vi "HFRR ADV v012 new software.vi"() -> ()   [LabVIEW 2025]
uses:
  <vilib>/picture/picture.llb/imagedata.ctl
  src/Support Vi/Auto Start enum.ctl
  src/CAMERA CODE/CAMERA LIVE FEED ENUM.ctl
  src/CAMERA CODE/POST ANALYSIS ENUM.ctl
  <vilib>/Utility/NIReport.llb/HTML Report Image Alignment.ctl
  9464fbe3-7a28-44f6-aba5-8c8738b059c4.vi
  65798b11-504e-4bc8-a248-6a605d2bfeff.vi
  e8a7d01f-49de-42c3-94d4-2c8624f58f4e.vi
  5efb8110-29bd-47d9-92d0-c4703c9d257e.vi
  c311699a-12ba-46ef-ac8f-427021fdbf06.vi
  b1c79803-6f73-4462-b675-f7b5eb88be7c.vi
  62610586-f3e3-47d7-ba3d-7d74a0c80884.vi
  25e8caaf-84ea-468e-9ff7-adb0e8b96af1.vi
  63a25930-3a94-42f5-b8a7-a5485c4ba60b.vi
  865355ac-209e-4fc1-945d-f9c41f79343a.vi
  8bf3357a-fd86-4b15-a53b-ddd460c8ef7b.vi
  8955922f-f541-41b3-8336-ee15e0ce1609.vi
  <vilib>/numeric/Random Number (Range) DBL.vi
  <vilib>/Analysis/baseanly.llb/Mean (DBL).vi
  <vilib>/Utility/error.llb/Trim Whitespace One-Sided.vi
  <vilib>/Instr/_visa.llb/VISA Configure Serial Port (Instr).vi
  Instance          10 41Saved   WinDucom--std ed hfrr-WO 2464 v02 .vi
  <vilib>/addons/control/pid/pid.llb/PID (DBL).vi
  Instance          23 41Saved   WinDucom--std ed hfrr-WO 2464 v02 .vi
  <vilib>/Utility/NIReport.llb/Append Image to Report (path wrap).vi
  <vilib>/printing/OpenHTMLReport.llb/Open HTML Report in Browser (Refnum).vi
  <vilib>/Utility/NIReport.llb/Append Report Text (str wrap).vi
  Instance          11 41Saved   WinDucom--std ed hfrr-WO 2464 v02 .vi
  Instance           6 41Saved   WinDucom--std ed hfrr-WO 2464 v02 .vi
  <vilib>/Utility/NIReport.llb/NI_report.lvclass
  <vilib>/addons/control/pid/NI_PID_pid.lvlib
  Instance          22 41Saved   WinDucom--std ed hfrr-WO 2464 v02 .vi
  Instance          25 41Saved   WinDucom--std ed hfrr-WO 2464 v02 .vi
  <vilib>/NI Modbus.llb/MB Serial Master Query Read Input Registers (poly).vi
  Instance          35 41Saved   WinDucom--std ed hfrr-WO 2464 v02 .vi
  Instance          38 41Saved   WinDucom--std ed hfrr-WO 2464 v02 .vi
  <vilib>/Utility/NIReport.llb/NI_ReportGenerationCore.lvlib
  <vilib>/Analysis/NI_AALPro.lvlib
  <vilib>/Analysis/NI_AALBase.lvlib
  kernel32.dll
  <vilib>/measure/NI_MABase.lvlib
  <vilib>/NI Modbus.llb/MB Serial Master Query Write Single Register (poly).vi
  <vilib>/ptbypt/NI_PtbyPt.lvlib
panel:
  out "Status":dbl[](array[numeric])
  out "Calibrated Voltage Value":dbl[](array[numeric])
  out "1D stroke":dbl[](array[numeric])
  out "Calibration 1.2":dbl
  out "Calibration 1.0":dbl
  out "Calibration 0.8":dbl
  out "Calibration 0.6":dbl
  out "Calibration 0.4":dbl
  out "Calibration 0.2":dbl
  out "LVDT STROKE  Calibration":dbl
  in  "Continue Stroke step 9":bool
  in  "Step 7 Back":bool
  out "Boolean":bool
  out "Read Humidity":string
  out "LVDT STROKE":dbl
  out "AmbRaw":dbl
  out "SampleRaw":dbl
  out "Kd":dbl
  out "Ki":dbl
  out "Kp":dbl
  out "Active Error Code":dbl
  out "Vpp":dbl
  out "Dac Status":dbl
  out "Ambient Temperature":dbl
  out "Current Duty Cycle":dbl
  out "Target Sample Temperature":dbl
  out "Sample Temperature":dbl
  in  "Add up Stroke":dbl=0.03
  out "START TEMP":bool
  in  "Command":string
  out "Due read":string
  out "UNI READ":string
  in  "STROKE":dbl[](array[numeric])=[0.1, 0.2, 0.3, 0.4, 0.5, 0.6, 0.7, 0.8, 0.9, 1.0, 1.1, 1.2]
  in  "1,2":dbl=1.1278
  in  "1.1":dbl=1.0761
  in  "1.0":dbl
  in  "0.9":dbl=0.9543
  in  "0.8":dbl
  in  "0.7":dbl=0.8122
  in  "0.6":dbl
  in  "0.5":dbl=0.639
  in  "0.4":dbl=0.5425
  in  "0.3":dbl=0.4226
  in  "0.2":dbl=0.2961
  in  "0.1":dbl=0.1677
  in  "calibration values":dbl[](array[numeric])=[0.1677, 0.2961, 0.4226, 0.5425, 0.639, 0.737, 0.8122, 0.864, 0.9543, 1.0177, 1.0761, 1.1278]
  out "prev_vc_cmd":dbl
  out "integral_accumulator_in":dbl
  out "prev_error":dbl
  in  "startup_cmd":dbl=400.0
  in  "min_amplitude":dbl
  in  "max_amplitude":dbl=1300.0
  in  "max_step_change":dbl=45.0
  in  "kd":dbl=40.0
  in  "ki":dbl=300.0
  in  "kp":dbl=1000.0
  in  "dt":dbl=0.05
  out "output Vpp":dbl
  out "error out 9":errorcluster
  out "LVDT MIN":dbl
  out "LVDT MAX":dbl
  out "LVDT Peak":dbl
  out "pizo raw":dbl
  out "Friction":dbl
  out "cof 2":dbl
  in  "main tab sub":enum32{"Page 1", "Page 2"}(tab)
  out "About":cluster{"About Display":string}={"About Display"="Software Version : Lab IQ\\WO 2472\\ v02\n\nRelease Period    : May 2026  "}
  in  "Info":bool
  in  "Quit":bool
  out "Humidity Port":bool=TRUE caption="Port 2"
  out "Standard 2":string="ASTM D6079 TEST CONDITIONS"
  out "powstat":bool caption="Power Status"
  out "Test \nStatus":bool caption="Test Status"
  out "Port 3":bool=TRUE caption="Port 1"
  out "Port 1a":bool caption="Port 1 a"
  out "Port 4":bool=TRUE caption="Port 2"
  out "Port 2a":bool caption="Port 2 a"
  in  "Main Dashboard Buttons":T1(radio) caption="Radio Buttons - Customizable"
  out "Time Stamp":string
  in  "Main Tab":T2(tab)
  out "Service Password Log":string="Incorrect Password"
  in  "Password 3":cluster{"Service Password":string}
  in  "Headen Service Button":bool
  in  "Sign In":bool
  in  "USER ID":string
  in  "USERNAME":string
  out "Auto Scar Check":cluster{"String 2":string}
  in  "Calibration":bool
  in  "Auto":bool
  in  "test time":dbl=75.0 caption="TEST DURATION" min=1.0 max=75.0 step=1.0
  in  "Set Rh":dbl=53.0 caption="HUMIDITY" min=53.0 max=53.0 step=1.0
  in  "Set Temp":dbl=60.0 caption="TEMPERATURE" min=40.0 max=150.0 step=1.0
  in  "Set Strk":dbl=1.0 caption="STROKE LENGTH" min=1.0 max=1.0 step=1.0 format="%.3f"
  in  "NORMAL LOAD":dbl=2.0 caption="APPLIED LOAD" min=1.0 max=10.0 step=1.0
  in  "Set Hz":dbl=50.0 caption="FREQUENCY" min=50.0 max=50.0 step=50.0 format="%.1f"
  out "Standard":string="ASTM D6079 TEST CONDITIONS"
  in  "FILE":string caption="FILE NAME"
  in  "Fuel Discription :":string caption="FLUID DESCRIPTION"
  in  "Batch Ref Num :":string caption="BATCH REF NO"
  in  "Remarks :":string caption="REMARKS"
  in  "tested by":string caption="TESTED BY"
  in  "Operator ID":string caption="OPERATOR ID"
  in  "TEST STANDARD":T3(ring)
  in  "Save & Continue":bool
  in  "Calibration 2":enum32{"Main", "Page 2"}(tab)
  in  "Cal Password":string
  out "Wrong Password":string="Wrong Password Entered"
  out "Time Remaining":dbl min=0.0 max=6000.0 step=0.01 format="%<%M:%S>t"
  in  "EVENT LOG":string="4:36:36 PM       Temperature trip enabled\n4:59:03 PM       Test started  — ASTM D6079-25"
  in  "Single/Multiple":enum32{"Single ", "Multiple"}(radio)=enum."Multiple" caption="Radio Buttons - Customizable"
  in  "Single - Graph":u16(ring) items=["Co-efficient of Friction", "Frictional Force ( N )", "ECR ( % )", "Temperature ( Deg C )", "Humidity ( %RH )", "Stroke ( mm )"]
  in  "Num/Graph":enum32{"Numeric Display", "Graph Display"}(radio) caption="Radio Buttons - Customizable"
  in  "Reset Graph":bool
  in  "Main Tab Display":T4(tab)
  out "COF 3":dbl min=0.0 max=1.0 step=0.001 format="%.3f"
  out "measured_stroke":dbl format="%.3f"
  in  "FRICVALZ 4":bool
  out "Set Stroke:":dbl
  out "Set Frequency:":dbl
  out "Set Humidity:":dbl
  out "Set Temperature:":dbl
  in  "Humidity":bool
  out "Horizontal Slider Control":dbl(slide) min=0.0 max=100.0 scale=0.0..75.0
  in  "Heater Button":bool
  out "HEATER":bool
  out "Humidity ( %RH )":dbl caption="Humidity 3" format="%.1f"
  out "AIR TEMP":dbl caption="Air Temperature  ( °C )" min=0.0 max=150.0 step=1.0 format="%.1f"
  out "Frequency ( Hz )":dbl=50.0 caption="Frequency" min=10.0 max=250.0 step=0.1 format="%.2f"
  out "Stroke 2":dbl=1.0 caption="Stroke" format="%.3f"
  out "TEMP":dbl min=0.0 max=150.0 step=1.0 format="%.1f"
  out "ecr 3":dbl min=0.0 max=100.0 step=1.0
  out "FF 3":dbl min=0.0 max=12.0 step=0.01 format="%.3f"
  out "Hum":dbl=34.66389660208565 min=0.0 max=150.0 step=1.0
  out "Stroke 4":dbl=1.0 caption="Stroke" format="%.3f"
  out "Stroke ( mm )":cluster{"y":dbl, dbl, "y":dbl}(graph) caption="Waveform Chart - Light"
  out "Humidity ( %RH )":dbl(graph) caption="Waveform Chart - Light"
  out "Status 13":bool
  in  "Set Temp 2":dbl=65.0 caption="TRIP" min=20.0 max=150.0 step=1.0
  in  "trip1 8":bool
  in  "FRICVALZ 2":bool
  out "COF 2":dbl min=0.0 max=1.0 step=0.001 format="%.3f"
  out "Coefficient of Friction":dbl(graph) caption="Waveform Chart - Light"
  out "Electrical Contact Resistance ( % )":dbl(graph) caption="Waveform Chart - Light"
  out "FF 2":dbl min=0.0 max=12.0 step=0.01 format="%.3f"
  out "Frictional Force ( N )":dbl(graph) caption="Waveform Chart - Light"
  out "TEMP 2":dbl=34.66389660208565 min=0.0 max=150.0 step=1.0
  out "Temperature ( Deg C )":dbl(graph) caption="Waveform Chart - Light"
  out "Single":T5(tab)
  out "COF 4":dbl min=0.0 max=1.0 step=0.001 format="%.3f"
  out "Coefficient of Friction":dbl(graph) caption="Waveform Chart - Light"
  out "FF 4":dbl min=0.0 max=12.0 step=0.01 format="%.3f"
  in  "FRICVALZ 3":bool
  out "Frictional Force ( N )":dbl(graph) caption="Waveform Chart - Light"
  out "Electrical Contact Resistance ( % )":dbl(graph) caption="Waveform Chart - Light"
  out "TEMP 3":dbl=34.66389660208565 min=0.0 max=150.0 step=1.0
  out "Temperature ( Deg C )":dbl(graph) caption="Waveform Chart - Light"
  out "Hum 2":dbl=34.66389660208565 min=0.0 max=150.0 step=1.0
  out "Humidity ( %RH )":dbl(graph) caption="Waveform Chart - Light"
  out "Stroke 3":dbl=1.0 caption="Stroke" format="%.3f"
  out "Stroke ( mm )":cluster{"y":dbl, dbl, "y":dbl}(graph) caption="Waveform Chart - Light"
  out "Test Duration Display":string
  in  "Test Duration Status":dbl(slide) scale=0.0..100.0
  in  "RUN":bool
  in  "Auto Start Test":bool caption="RUN"
  out "Auto Scar Check  2":cluster{"String 2":string}
  in  "Magnification len live scar":string(combo)="5x" caption="MAGNIFICATION LEVEL"
  in  "FILE 3":string(combo) caption="FILE NAME"
  in  "SCAR MEASURMENT":enum32{"Auto Scar", "Manual Scar"}(radio)=enum."Manual Scar" caption="Radio Buttons - Customizable"
  in  "Cap Live Image":bool caption="Save Image"
  out "Zoom Factore":dbl format="%#.0f"
  in  "OUT":bool
  in  "In":bool
  in  "Confirm Measrurement":bool
  in  "Magnification :":string(combo)="5x"
  in  "Open Image":bool
  in  "Test File List :":string(combo)
  in  "Calibration Tab":enum32{"Measrument", "Calibrate"}(tab)
  out "Major Axis":dbl
  out "Minor Axis":dbl
  out "Average":dbl
  in  "Back Square":bool
  out "10x Gain":dbl
  out "5x Gain":dbl
  in  "Actual (µm)":dbl=1.0 caption="Actual (mm)" format="%.6f"
  out "Measurment (mm)":dbl caption="mm" format="%.3f"
  in  "Save Change":bool caption="Save Cal"
  in  "change Gain":bool
  in  "Calibrate":bool
  in  "Resize Tool":bool
  in  "Fit to Screen Tool":bool
  in  "ROI Color Tool":bool
  in  "Clear ROI Tool":bool
  in  "Rectangle Tool":bool
  in  "Pan Tool":bool
  in  "line tool":bool
  in  "Frequency":bool
  in  "Sample Temperature":bool
  in  "Stroke":bool
  in  "Humidity":bool
  in  "Air Temperature":bool
  in  "Tab Control 2":T6(tab)=enum."Humidity"
  in  "rstv2":bool
  out "Coefficient Of Friction":cluster{dbl[], dbl[]}[](graph)
  out "КОФ1":dbl caption="COF1 :" min=0.0 max=200.0 step=0.1 format="%.3f"
  out "КОФ2":dbl caption="COF2 :" min=0.0 max=200.0 step=0.1 format="%.3f"
  out "КОФ3":dbl caption="COF3 :" min=0.0 max=200.0 step=0.1 format="%.3f"
  out "КОФ4":dbl caption="COF4 :" min=0.0 max=200.0 step=0.1 format="%.3f"
  in  "RSTV1 3":bool
  out "Air Temperature  ( °C )":cluster{dbl[], dbl[]}[](graph)
  in  "RSTV1 2":bool
  out "Humidity ( %RH )":cluster{dbl[], dbl[]}[](graph)
  in  "RSTV1 4":bool
  out "Stroke ( mm )":cluster{dbl[], dbl[]}[](graph)
  out "КОФ2 5":dbl caption="Stroke 4 :" min=0.0 max=200.0 step=0.1 format="%.3f"
  out "КОФ2 4":dbl caption="Stroke 3 :" min=0.0 max=200.0 step=0.1 format="%.3f"
  out "КОФ2 3":dbl caption="Stroke 2 :" min=0.0 max=200.0 step=0.1 format="%.3f"
  out "КОФ2 2":dbl caption="Stroke 1:" min=0.0 max=200.0 step=0.1 format="%.3f"
  out "CP2":dbl=nan min=0.0 max=200.0 step=0.1 format="%.3f"
  out "CP1":dbl=nan min=0.0 max=200.0 step=0.1 format="%.3f"
  in  "RST CP":bool
  out "Sample Temperature ( °C )":cluster{dbl[], dbl[]}[](graph)
  in  "RST CP 2":bool
  out "XY Graph 13":cluster{dbl[], dbl[]}[](graph)
  out "Frequency ( Hz )":cluster{dbl[], dbl[]}[](graph)
  in  "RST CP 3":bool
  out "Air Temp ( °C ) vs Humidity ( % RH )":cluster{dbl[], dbl[]}[](graph)
  in  "OPEN 1":bool
  out "String Control 2":string="  "
  out "String Control":string
  out "String Control 7":string
  in  "OPEN 4":bool
  out "String Control 8":string=" "
  in  "OPEN 2":bool
  out "String Control 3":string
  out "String Control 4":string=" "
  in  "OPEN 3":bool
  out "String Control 6":string=" "
  out "String Control 5":string
  in  "Coefficient Of Friction":bool
  in  "OPEN":bool
  in  "Main Calibration Tab":T7(tab)
  in  "Calibration Selection":T8(radio) caption="Radio Buttons - Customizable"
  in  "Main Stroke Tab":T9(tab)
  in  "Continue Stroke":bool
  in  "Back Stroke":bool
  in  "Step 2 Back":bool
  in  "Continue Stroke step 2":bool
  in  "Step 3 Back":bool
  in  "Continue Stroke step 3":bool
  in  "Step 4 Back":bool
  in  "Continue Stroke step 4":bool
  in  "Step 5 Back":bool
  in  "Continue Stroke step 5":bool
  in  "Step 6 Back":bool
  in  "Continue Stroke step 6":bool
  in  "Back Stroke step 7":bool
  in  "Continue Stroke step 7":bool
  in  "Stroke Test Complete":T10(tab)
  out "MOVE CARRIAGE TO":dbl caption="mm" format="%.1f"
  out "1.2":bool
  out "1.0 2":bool
  out "0.8 2":bool
  out "0.6 2":bool
  out "0.4 2":bool
  out "0.2 2":bool
  out "0.2mm":bool
  out "0.4 mm":bool
  out "0.6 mm":bool
  out "0.8mm":bool
  out "1.0 mm":bool
  out "1.2 mm":bool
  in  "Back Stroke step 8":bool
  in  "Continue Stroke step 8":bool
  in  "Back Stroke 8":bool
  in  "Accept & Save":bool
  out "Point 6 - 1.2 mm":bool caption="CONFIRMED"
  out "Point 5 - 1.0 mm":bool caption="CONFIRMED"
  out "Point 4 - 0.8 mm":bool caption="CONFIRMED"
  out "Point 3 - 0.6 mm":bool caption="CONFIRMED"
  out "Point 2 - 0.4 mm":bool caption="CONFIRMED"
  out "Point 1 - 0.2 mm":bool caption="CONFIRMED"
  in  "Tab Control 5":T11(tab)
  in  "message":string="*Entered password is wrong"
  in  "Password 2":string caption="Password (Advance Setting)"
  in  "EDIT 2":bool
  in  "Language Selection":enum16{"English", "Russian"}(ring)
  in  "SrvM CP 2":bool caption="Reset calibrate\n password"
  in  "SrvM CP":bool caption="Reset calibrate\n password"
  in  "Password":string
  in  "SAVE":bool
  in  "File Path":path=path "C:/LAB-IQ-NXT 2010/1582/1582" caption="File path"
  in  "EDIT":bool
  out "AIR TEMPERATURE  Calibration Error":dbl=1.0 caption="Air Temperature :" min=0.0001 max=100.0 step=0.0001
  out "TEMPERATURE  Calibration Error":dbl=1.0 caption="Temperature :" min=0.0001 max=100.0 step=0.0001
  out "HUMIDITY  Calibration Error":dbl=1.0 caption="Humidity :"
  out "DISPLACEMENT  Calibration Error":dbl=1.0255 caption="Displacement :"
  out "STROKE Calibration Error":dbl=700.0 caption="Stroke Gain :"
  out "FRIC. FORCE Calibration Error":dbl=3.7633 caption="Frictional Force :" min=0.0001 max=100.0 step=0.0001
  in  "AIR TEMP INTERCEPT: 2":dbl=-2.9906 caption="Air Temperature Intercept:" format="%.4f"
  in  "AIR TEMP INTERCEPT:":dbl caption="Air Temperature Intercept :" format="%.4f"
  in  "TEMP INTERCEPT: 2":dbl=-2.9906 caption="Temperature Intercept :" format="%.4f"
  in  "TEMP INTERCEPT:":dbl caption="Temperature Intercept :" format="%.4f"
  in  "AIR TEMPERATURE : 2":dbl=57.9984 caption="Air Temperature :" min=0.0001 max=100.0 step=0.0001 format="%.4f"
  in  "AIR TEMPERATURE :":dbl=1.0 caption="Air Temperature :" min=0.0001 max=100.0 step=0.0001 format="%.4f"
  in  "TEMPERATURE : 2":dbl=57.9984 caption="Temperature :" min=0.0001 max=100.0 step=0.0001 format="%.4f"
  in  "TEMPERATURE :":dbl=1.0 caption="Temperature :" min=0.0001 max=100.0 step=0.0001 format="%.4f"
  in  "HUMIDITY: 2":dbl=1.0 caption="Humidity :" min=0.95 max=1.05 step=0.001 format="%.2f"
  in  "HUMIDITY:":dbl=1.0 caption="Humidity :" min=0.95 max=1.05 step=0.01 format="%.2f"
  in  "DISPLACEMENT : 4":dbl=0.88 caption="Displacement :" min=0.5 max=1.8 step=0.01 format="%#.2f"
  in  "DISPLACEMENT :":dbl=1.0255 caption="Displacement :"
  in  "STROKE GAIN : 2":dbl=900.0 caption="Stroke Gain :" min=500.0 max=1500.0 format="%#.1f"
  in  "STROKE GAIN :":dbl=700.0 caption="Stroke Gain :"
  in  "FRIC. FORCE : 2":dbl=1.0 caption="Frictional Force :" min=0.95 max=1.05 step=0.0001 format="%.2f"
  in  "FRIC. FORCE :":dbl=3.7633 caption="Frictional Force :" min=0.0001 max=100.0 step=0.0001 format="%.4f"
  in  "Tab Control 7":T12(tab)
  in  "S.NO":string="1333"
  in  "Standard Slip Gauge (mm)":dbl
  out "String 26":string="Rh"
  out "String 13":string="Rh"
  out "String 5":string="N"
  out "String 3":string="Hz"
  out "Time slide":dbl(slide)=70.0 scale=0.0..2500.0
  in  "ENTER THE NEW PASSWORD":string caption="Enter The New Password"
  in  "ENTER CURRENT PASSWORD":string caption="Enter Current Password"
  in  "Camera Port :":string(combo)="cam0"
  in  "C3 :":refnum<visa-resource-name>="COM8"
  out "Port 2 Error":errorcluster={"status"=TRUE, "code"=-1073807343, "source"="Property Node (arg 1) in VISA Configure Serial Port (Instr).vi->Winducom 2010--std ed hfrr-wo1768-V18.vi"}
  out "Port 1 Error":errorcluster={"status"=TRUE, "code"=-1073807343, "source"="Property Node (arg 1) in VISA Configure Serial Port (Instr).vi->Winducom 2010--std ed hfrr-wo1768-V18.vi"}
  in  "CH-HUMIDITY DRY":u16=3 caption="Ch-Humidity Wet:" max=7 step=1
  in  "CH-HUMIDITY WET":u16=4 caption="Ch-Humidity Dry:" max=7 step=1
  in  "CH-HEATER":u16=2 caption="Ch-Heater:" max=7 step=1
  in  "CH-POWER -":u16=1 caption="Ch-Power -:" max=7 step=1
  in  "CH-POWER +":u16 caption="Ch-Power +:" max=7 step=1
  out "String 4":string
  in  "Prog Due":bool
  in  "Prog Uno":bool
  in  "Com Port 2":refnum<visa-resource-name>="COM7" caption="C2 :"
  in  "Com Port 1":refnum<visa-resource-name>="COM5" caption="C1 :"
  in  "SAVE 2":bool
  in  "Additional Parameter":T13(tab)
  out "CAMERA ROI MIN TEMP":bool
  in  "CAMERA ROI MAX TEMP":bool
  out "LIVE FEED MIN TEMP":bool
  in  "LIVE FEED MAX TEMP":bool
  in  "Temperature Off Command":bool
  in  "Temperature On Command":bool
  in  "Humidity Off Command":bool
  in  "Humidity On Command":bool
  out "Elapsed time":dbl caption="Elapsed Time" min=0.0 max=6000.0 step=0.01 format="%.2f"
  in  "Remaining Time":dbl min=0.0 max=180000.0 step=0.0001 format="%<%H:%M:%S>t"
  out "Auto Start Temp":bool
  out "Auto stop temp":bool
  in  "TestCompFlg":bool
  out "StartFlg":bool
  in  "Start Time":bool
  in  "sign in temp":bool
  in  "manual temp log":bool
  in  "Reach point temp":bool
  in  "Manual Humididty Reached":bool
  out "Humidity temp":dbl
  in  "Test ID":string
  in  "Reach point Humidity":bool
  in  "error in (no error) 2":errorcluster
  out "Instrument Status":bool=TRUE caption="Load COM Status"
  in  "Heater Trip Temp":bool
  out "String 41":string=":-@(Paltro : HIGH FREQUENCY RECIPROCATORY TEST RIG    DEFINITON FILE )      "
  out "Service Password enable":bool
  out "TEST FILE NAM,E SAVED":bool
  out "error out 6":errorcluster
  out "error out 7":errorcluster
  out "error out 8":errorcluster
  in  "Ambient Humidity :":dbl format="%.1f"
  out "Camera List":string
  out "Image path  2":path caption="selected path"
  out "100x gain":dbl
  out "Pixel Value":dbl
  in  "Enum - Selector":T14
  out "Image path":path
  out "Error":errorcluster={"status"=TRUE, "code"=-1073807343, "source"="Property Node (arg 1) in VISA Configure Serial Port (Instr).vi->Winducom 2010--std ed hfrr-wo1768-V18.vi"}
  out "Bytes at Humidity Port":dbl
  in  "Com Port 4":refnum<visa-resource-name>="COM7" caption="COM Port Humidity :"
  in  "String 11":string
  in  "WriteHumidity":string[](array[string])
  out "LastCom":string
  in  "Write S":bool
  out "STALL :":string
  out "CURRENT :":string
  out "DEHUM :":string
  out "FAN_OUT :":string
  out "FAN_IN :":string
  out "PUMP :":string
  out "AMB_T :":string
  out "AMB_RH :":string
  out "T :":string
  out "RH :":string
  out "SET :":string
  out "STATE :":string
  out "RH Numeric:":dbl
  out "COM Status":bool=TRUE caption="Load COM Status"
  in  "Tab Control 6":enum32{"Data", "Sensor"}(tab)=enum."Sensor"
  out "Respose From Server":string
  out "standard output":string
  out "SinglePoint":string
  in  "JSON Check String":string="\"Stored\": true"
  in  "JSONH Check String":string="\"Stored\": true"
  out "standard output 2":string
  in  "Sensor Information":string[][](array[string])=[["Sensor Name", "Sensor Model Number", "Sensor Run time Hours", "Sensor State"], ["Normal Load Sensor", "MPF-AC20-X3U791", "", ""], ["Frictional Force Sensor", "MPF-AC20-X3U792", "", ""], ["Temperature Sensor", "MPF-AC20-X3U793", "", ""], ["Speed Sensor", "MPF-AC20-X3U794", "", ""], ["LVDT Sensor", "MPF-AC20-X3U795", "", ""], ["Vibration Sensor ", "MPF-AC20-X3U796", "", ""]]
  out "Respose From Server 2":string
  in  "Total No. of Tests":dbl
  in  "Upld AR":bool
  in  "Sensor File Name":string="JSON_Health.JSON"
  in  "Run test 3":bool
  in  "Sen.Upload Rate (s)":dbl=5.0 min=0.5 max=5.0 step=0.5 format="%.1g"
  in  "Upld AR 2":bool
  in  "Path":path=path "C:/LAB-IQ-NXT"
  in  "Data File Name":string="JSON_Single_Point.JSON"
  in  "Model No":string="MD987654325"
  in  "Serial No":string="HFRR2391"
  in  "Secret Key":string="22gKHnAGFaJhuNtaR9srYhcD6RQR8M7Zp2xk4ssPTuwGqWUBv7WxW7cXAFkFFbns"
  in  "Upload Rate (s)":dbl=1.0 min=0.5 max=5.0 step=0.5 format="%.1g"
  out "Test Standard":string
  out "error out 5":errorcluster
  out "after substring":string
  out "before substring 2":string
  in  "Temperature after test 3":dbl caption="Temp After Test" format="%#_5g"
  in  "Humidity after test 3":dbl caption="Humidity After Test" format="%#_5g"
  out "autostrtflg":bool
  out "airtempflg":bool
  out "z_measure":dbl
  out "Read String":string
  out "Waveform Graph 5":dbl[](graph)
  out "Waveform Chart 3":dbl[](graph)
  out "set temp old":dbl
  out "Error Code":errorcluster
  in  "Rd":bool
  out "String 10":string
  in  "Length 2":i16=16 caption="Set" min=1 max=60 step=1
  out "path 2":path
  out "image data":T15
  out "new picture":picture
  out "error out 2":errorcluster
  out "String Indicator 4":string
  out "String Indicator 3":string
  in  "OPEN 5":bool
  out "string1 5":string
  out "String 49":string="Tested by"
  out "String 48":string="Sample ID "
  out "String 47":string="Tested date"
  out "String 46":string="S.NO"
  out "test by 2":string
  in  "ISO : WS1.4":enum32{"Page 1", "Page 2"}(tab)
  in  "Save Results":bool
  out "String 23":string="ISO : WS1.4"
  out "Rh After":dbl min=0.0 max=100.0 step=1.0 format="%.1f"
  out "Rh Before":dbl min=0.0 max=100.0 step=1.0 format="%.1f"
  in  "Humidity before test":dbl min=0.0 max=100.0 step=1.0
  out "AVP":dbl=0.0032746494993313616 format="%.3f"
  in  "MWSD":dbl
  out "WS1.4":dbl format="%1.2f"
  in  "HCF":dbl min=0.0 max=10000.0 step=0.01 format="%.2f"
  in  "Temperature before test":dbl=1.0 caption="Temp before test" min=1.0 max=100.0 step=0.1 format="%.1f"
  in  "Humidity after test":dbl=1.0 min=1.0 max=100.0 step=1.0
  in  "Temperature after test":dbl=1.0 caption="Temp after test" min=1.0 max=100.0 step=0.1 format="%.1f"
  out "WS1.4 2":dbl caption="WS1.4" format="%#_5g"
  out "HCF 2":dbl caption="HCF" format="%#_5g"
  out "AVP 2":dbl caption="AVP" format="%#_5g"
  out "MWSD 2":dbl caption="MWSD" format="%#_5g"
  out "Temperature after test 2":dbl caption="Temp after test" format="%#_5g"
  out "Humidity after test 2":dbl caption="Humidity after test" format="%#_5g"
  out "Temperature before test 2":dbl caption="Temp before test" format="%#_5g"
  out "Humidity before test 2":dbl caption="Humidity before test" format="%#_5g"
  out "temp_@Rh sensor":string
  out "refresh flag":bool
  out "Air temp":string
  in  "hide controller":enum32{"Hidden", "controllers"}(tab)=enum."controllers"
  in  "UUID":string caption="UUID    :"
  in  "FLAG 4":dbl min=0.0 max=999999999.0 step=0.25 format="%.2f"
  out "START 3":dbl format="%.1f"
  in  "FLAG 2":dbl min=0.0 max=999999999.0 step=0.25 format="%.2f"
  out "JSON string":string
  out "Sensor Health JSON string":string
  out "run replace":bool
  out "cof":dbl caption="Frictional Torque" format="%.2f"
  out "time":dbl caption="Time \nRemaining"
  out "SEN.RUN HRS":dbl
  out "Json St Flg":bool
  out "Json End Flg":bool
  out "temp_st":string
  out "sp_st":string
  out "FF STATE":i32
  out "nlstate":string
  out "ffstate":string
  out "nl_st":string
  out "ff_st":string
  in  "in":string[](array[string])=["", "", "", "", "", "", ""]
  out "out":string[](array[string])=["Sensor State", "", "", "", "", "", ""]
  out "SinglePoint  2":string
  out "Sensor name":string[](array[string])
  out "model num":string[](array[string])
  out "run time":string[](array[string])
  out "state":string[](array[string])
  out "state1":string[](array[string])
  out "T cycle":dbl caption="TOTAL\nTIME"
  in  "Length":i16=16 caption="Set" min=1 max=60 step=1
  out "acq 2":bool
  out "Stroke Ln 2":string
  out "St Str":string
  out "run":string[](array[string])
  out "run hrs":string
  in  "tfalg":dbl
  out "Temp":dbl caption="Pin temp"
  in  "yflag":dbl
  in  "zflag":dbl
  out "zflag 2":dbl
  out "SENSOR TIME":dbl
  out "TEMP STATE":i32
  out "NL STATE":i32
  in  "FLAG":dbl min=0.0 max=999999999.0 step=0.25 format="%.2f"
  out "START 2":dbl format="%.1f"
  out "SENSOR TIME  2":dbl
  out "Rt 3":bool
  out "Rt":bool
  out "Rt 2":bool=TRUE
  in  "Reset 4":bool caption="Reset"
  in  "tmpchk":bool
  out "Temp ini":dbl min=0.0 max=150.0 step=1.0
  in  "wait":u32=1000
  out "humid":string
  out "Ser Led":bool
  in  "Send":bool
  out "Humidity Str Rec":string
  in  "Humidity Str Send":string="stop"
  out "visa due":string(combo)="COM63" caption="Visa Module 2 ( Due )"
  in  "Tab Control":T16(tab)
  out "Calibration Tare Value":dbl
  out "Calibration Tare":bool
  out "Position Measurment Temp":dbl
  in  "Info Square":bool
  out "String 43":string="mm"
  in  "Home 8":bool
  in  "Home 9":bool
  out "String 18":string="min"
  out "String 22":string="min"
  out "String 17":string="Timer"
  in  "Samplingtime 2":dbl=0.5 caption="Save Dwell" min=0.1 max=600.0 step=0.1 format="%.1g"
  out "String 21":string="Sec"
  in  "RST FF":bool
  in  "RSTCOF 3":bool
  in  "RST TEMP":bool
  in  "RSTCOF":bool
  in  "Home":bool caption="Password"
  in  "Configure":bool caption="Password"
  in  "Analysis 2":bool caption="Password"
  in  "service 3":bool caption="Password"
  in  "EXIT 2":bool
  in  "GRAY SCALE INTERCHANGE":enum32{"GRAY IMAGE", "RGB IMAGE"}(radio)=enum."RGB IMAGE"
  in  "Lubrication System COM Port :":refnum<visa-resource-name>="COM9" caption="Ambient Temperature COM Port:"
  in  "Com Port 3":refnum<visa-resource-name>="COM4" caption="Port 3"
  in  "STOP 2":bool
  out "Upload \nConfirmed 2":bool caption="Health"
  out "Upload \nConfirmed":bool caption="Data"
  out "AR Led":bool caption="AR"
  in  "Air Temp vs Humidity":bool
  in  "autostart":bool caption="RUN"
  in  "SetTemp 2":dbl=23.0 caption="Set" min=1.0 max=26.0 step=1.0
  out "autostart 2":string
  out "String 14":string
  out "TK4 status":bool=TRUE caption="Air Status"
  in  "Heater":bool
  out "Amb temp":dbl caption="Air Temperature" min=0.0 max=150.0 step=1.0 format="%.1f"
  out "SetTemp":dbl=23.0 caption="Set" min=20.0 max=26.0 step=1.0
  in  "Engage":bool
  out "Countdown 2":dbl caption="Present ( Sec )" min=1.0 max=6000.0 step=1.0
  in  "Countdown":dbl=1.0 caption="Count down ( Sec )" min=1.0 max=6000.0 step=1.0
  out "COF - filtered":dbl min=0.0 max=200.0 step=0.1 format="%.2f"
  in  "% Humidity":dbl=35.0 min=1.0 max=100.0 step=1.0
  out "Peak - Peak 2":dbl
  out "COF":dbl=100.0 min=0.0 max=200.0 step=0.1 format="%.1f"
  out "act save time":dbl=3561152582.7339997 format="%.2f"
  out "acq timer":dbl=3614575087.823 format="%.2f"
  out "Cycles elapsed":i32=5
  in  "Save":bool
  out "cyclecount":i32
  out "speedop":dbl min=0.0 max=999999999.0 step=0.25 format="%.2f"
  out "cmp":i32
  in  "OPEN 6":bool
  out "freq1":dbl format="%_4f"
  out "freq2":dbl format="%_4f"
  out "freq3":dbl format="%_4f"
  out "sample1":dbl format="%_4f"
  out "sample2":dbl format="%_4f"
  out "sample3":dbl format="%_4f"
  out "String 6":string="  "
  in  "String 7":string="  "
  out "String 12":string="  "
  out "String 8":string="  "
  out "Numeric 13":i32
  out "Numeric 12":i32
  out "Numeric 11":i32
  out "Numeric 8":i32
  in  "Ref B Scar Value :":string caption="Reference Fluid Information"
  in  "Ref B Test Date :":string caption="Reference Fluid Information"
  in  "Ref A Scar Value :":string caption="Reference Fluid Information"
  in  "Image Path":path
  in  "Wear Scar Y":dbl caption="Wear Scar Minor Axis ( Microns )" format="%#_5g"
  in  "Wear Scar X":dbl caption="Wear Scar Major Axis ( Microns )" format="%#_5g"
  in  "Print 2":bool caption="Печать"
  in  "Ref A Test Date :":string caption="Reference Fluid Information"
  out "XY Graph 17":cluster{dbl[], dbl[]}[](graph)
  in  "Print 3":bool caption="Печать"
  in  "Select File Type":enum16{"xlx", "csv", "txt"}(ring)
  out "s.NO":string caption="S.NO"
  in  "Export":bool
  out "Test Date":string caption="Tested date"
  out "Tested by":string
  out "Sample ID":string
  in  "OK Button 16":bool
  out "String Indicator":string
  out "String Indicator 2":string
  in  "OK Button 17":bool
  out "Selected Printer":string="Microsoft XPS Document Writer"
  in  "Select Printer 3":i32 caption="Select Printer"
  out "System Configured Printers 2":string[](array[string])=["Microsoft XPS Document Writer", "Fax", "CutePDF Writer", "\\\\192.168.1.28\\RICOH Aficio MP 2352 PCL 6"] caption="System Configured Printers"
  out "TITTLE":string caption="Tittle"
  in  "Sample ID  5":string caption="Fuel S/N:"
  in  "Sample ID  4":string caption="Fuel Name:"
  in  "Sample ID  3":string caption="Fuel Type:"
  in  "Print":bool caption="Печать"
  in  "SPEED OUT:":dbl=1.0 caption="Speed Out:" min=0.0001 max=5.0 step=0.0001 format="%.4f"
  in  "Temperature before test 3":dbl caption="Temp Before Test" format="%#_5g"
  in  "Humidity before test 3":dbl caption="Humidity Before Test" format="%#_5g"
  out "Temperature after test 5":dbl caption="Temp Before Test" format="%#_5g"
  out "Temperature after test 4":dbl caption="Temp After Test" format="%#_5g"
  out "Humidity after test 4":dbl caption="Humidity After Test ( % Rh )" format="%#_5g"
  out "Humidity before test 4":dbl caption="Humidity Before Test ( % Rh )" format="%#_5g"
  in  "Tab Control 9":enum32{"Page 1", "Page 2"}(tab)
  out "Ref B Scar Value :":string caption="Reference Fluid Information"
  out "Ref B Test Date :":string caption="Reference Fluid Information"
  out "Ref A Scar Value :":string caption="Reference Fluid Information"
  out "Ref A Test Date :":string caption="Reference Fluid Information"
  out "XY Graph 16":cluster{dbl[], dbl[]}[](graph)
  out "TITTLE 4":string caption="Reference Fluid Information"
  out "Sample ID  7":string caption="Fuel Name :"
  out "Sample ID  6":string caption="Fuel Type :"
  out "Mean Wear ( microns) :":dbl format="%#.6f"
  out "Wear Scar Y ( microns ) :":dbl format="%#.6f"
  out "Length ( microns ) 2":dbl caption="Wear Scar X ( microns ) :" format="%#.6f"
  out "s.NO 2":string caption="Instrument  S.NO :"
  out "Test Date 2":string caption="Tested date :"
  out "Tested by 2":string caption="Tested by :"
  out "Sample ID  2":string caption="Sample ID :"
  out "TITTLE 2":string caption="File Name :"
  in  "EDIT 3":bool
  out "FF buffer":dbl[](graph)
  out "%  o/p":dbl
  out "sample4":dbl format="%_4f"
  out "freq 4":dbl format="%_4f"
  out "conststatus":dbl=10.0 min=0.0 max=200.0 step=1.0
  out "CP4":dbl=nan min=0.0 max=200.0 step=0.1 format="%.3f"
  out "CP3":dbl=nan min=0.0 max=200.0 step=0.1 format="%.3f"
  out "Boolean  4":bool=TRUE caption="Power Status"
  in  "Boolean BC T & BG 2":cluster{u32, u32}[](array[cluster])=[{3158064, 16250871}, {11918296, 8965631}]
  in  "GBG   2":u32(colorbox)=16250871 caption="Graph Background"
  in  "GFG  2":u32(colorbox)=8964095 caption="Graph Foreground"
  in  "GBG":u32(colorbox)=16250871 caption="Graph Background"
  in  "GFG":u32(colorbox)=8964095 caption="Graph Foreground"
  in  "Boolean BC T & BG":cluster{u32, u32}[](array[cluster])=[{3158064, 16250871}, {11918296, 8965631}]
  in  "SC  Text":u32(colorbox) caption="String Control Text"
  in  "SC BG 3":u32(colorbox)=16777215 caption="String Control BG"
  in  "NI BG 2":u32(colorbox)=13553358 caption="Numeric Indicator BG"
  in  "NI Text  2":u32(colorbox)=7105644 caption="Numeric Indicator Text"
  in  "NC Text":u32(colorbox)=3381759 caption="Numeric Control Text"
  in  "NC BG":u32(colorbox)=16777215 caption="Numeric Control BG"
  in  "Com flag":u32
  out "Gain path":string="C:\\Winducom 2010\\STD ED HFRR\\wo1768"
  out "String 45":string="S.NO"
  out "String 44":string
  out "error out 4":errorcluster
  out "concatenated string 2":string
  out "String 42":string
  out "error out 3":errorcluster
  out "STR":string
  out "gain":string
  out "export":string
  out "before substring":string
  out "output":string
  out "test by":string
  out "export 2":string
  out "export":string
  out "REMARKS 2":string="@WINDUCOM : RECIPROCATORY TEST RIG    DEFINITON FILE       \r  Sample ID :- , Load :-  2.00 N , Remarks :- , Date :- 05/11/2016, 06:04\r"
  out "data":string
  out "Boolean 3":bool
  out "concatenated string":string
  out "path":path
  out "String 40":string
  out "Boolean 2":bool=TRUE
  in  "Set Rh 2":dbl=50.0 caption="HUMIDITY" min=35.0 max=85.0 step=1.0
  out "String 39":string="WS1.4="
  out "String 38":string="HCF="
  out "String 37":string="MWSD="
  out "String 36":string="AVP ="
  out "String 35":string="Temp after test="
  out "String 34":string="Temp before test="
  out "String 33":string="Tested by"
  out "String 32":string="Sample ID "
  out "String 31":string="Tested date"
  out "String 30":string="Sample Design"
  out "path string":string
  out "String 29":string
  out "St. Line eqn : 2":string
  out "Numeric 10":i32
  out "Numeric 16":i32
  out "S 106":string="Off"
  out "S 105":string="On"
  out "S 104":string="Heater Off"
  out "S 103":string="Heater On"
  out "S 102":string="Ch-Humidity Dry:"
  out "S 101":string="Ch-Humidity Wet:"
  out "S 100":string="Ch-Heater:"
  out "S 99":string="Ch-Power -:"
  out "S 98":string="Ch-Power +:"
  out "S 97":string="Port 2"
  out "S 96":string="Port 1"
  out "S 95":string="Stroke Gain :"
  out "S 94":string="Displacement :"
  out "S 93":string="Stop"
  out "S 92":string="Run"
  in  "LAnguage":enum32{"Page 1", "Page 2"}(tab)
  out "S 91":string="Threshold"
  out "S 90":string="File path"
  out "S 89":string="Newtons ( N )"
  out "S 88":string="Change Calibrate Password"
  out "S 87":string="Enter The New Password"
  out "S 86":string="Enter Current Password"
  out "S 85":string="Password"
  out "S 84":string="Save Gain Constants"
  out "S 83":string="Air Temperature ( deg C )"
  out "S 82":string="TIME ( mins )"
  out "S 81":string="Relative Humidity ( Rh )"
  out "S 80":string="Sample TEMPERATURE ( Deg C)"
  out "S 79":string="Stroke"
  out "S 78":string="Air Temperature"
  out "S 77":string="mm"
  out "S 76":string="Stroke"
  out "S 75":string="WINDUCOM 2010 \\XXXX\\VX.XX\\MONTH YEAR"
  out "S 74":string="Frictional Force ( N )"
  out "S 73":string="Calibrate Parameter"
  out "S 72":string="Save Gain Constant"
  out "S 71":string="Edit Gain Constant"
  out "S 70":string="Humidity :"
  out "S 69":string="Air Temperature :"
  out "S 68":string="Speed Out:"
  out "S 67":string="Temperature :"
  out "S 66":string="Frictional Force :"
  out "S 65":string="ABOUT"
  out "S 64":string="Frictional  Force ( N )"
  out "S 63":string="Temperature ( Deg C)"
  out "S 62":string="Time ( mins )"
  out "S 60":string="Reset Graph"
  out "S 59":string="COF4"
  out "S 58":string="COF3"
  out "S 57":string="COF2"
  out "S 56":string="COF1"
  out "S 55":string="Frictional Force ( N )"
  out "S 54":string="Temperature"
  out "S 53":string="Coefficient Of Friction"
  out "S 52":string="Refresh"
  out "S 51":string="File 4"
  out "S 50":string="File 3"
  out "S 49":string="File 2"
  out "S 48":string="File 1"
  out "S 47":string="COMPARE FILES"
  out "S 46":string="SAVE RESULT"
  out "S 45":string="WS1.4"
  out "S 44":string="HCF"
  out "S 43":string="MWSD"
  out "S 42":string="AVP "
  out "S 41":string
  out "S 40":string
  out "S 39":string="Humidity after test="
  out "S 38":string="Humidity before test="
  out "S 37":string
  out "S 36":string="Rh Before"
  out "S 35":string="ISO : WS1.4"
  out "S 34":string="FRICTIONAL FORCE ( N )"
  out "S 33":string="Reset Graph"
  out "S 32":string="Data points"
  out "S 31":string="COEFFICIENT OF FRICTION"
  out "S 30":string="RUN"
  out "S 29":string="Test Status"
  out "S 28":string="Power"
  out "S 27":string="Engage"
  out "S 26":string="Present ( Sec )"
  out "S 25":string="Count down ( sec )"
  out "S 24":string="Sec"
  out "S 23":string="Save Dwell"
  out "S 22":string="Elapsed Time"
  out "S 21":string="min"
  out "S 20":string="Test duration"
  out "S 19":string="TIMER"
  out "S 18":string="OFF"
  out "S 17":string="Rh"
  out "S 16":string="HUMIDITY"
  out "S 15":string="Heater On"
  out "S 14":string="TEMPERATURE ( Deg C)"
  out "S 13":string="N"
  out "S 12":string="NORMAL LOAD"
  out "S 11":string="Hz"
  out "S 10":string="FREQUENCY"
  out "S 9":string="STOP"
  out "S 8":string="STAND BY"
  out "S 7":string="Remarks :"
  out "S 6":string="Sample ID :"
  out "S 5":string="File Name :"
  out "S 4":string="Acquire"
  out "S 3":string="EXIT"
  out "S 2":string="Winducom 2010"
  out "S":string="ENGLISH TITLES"
  out "Error Due":errorcluster={"status"=TRUE, "code"=-1073807343, "source"="Property Node (arg 1) in VISA Configure Serial Port (Instr).vi->Winducom 2010--std ed hfrr-wo1768-V18.vi"}
  out "Error Uno":errorcluster={"status"=TRUE, "code"=-1073807343, "source"="Property Node (arg 1) in VISA Configure Serial Port (Instr).vi->Winducom 2010--std ed hfrr-wo1768-V18.vi"}
  out "as":string
  out "bs":string="Rh After"
  out "as":string=" after test"
  out "bs":string="Temp"
  out "as":string=" before test"
  out "bs":string="Temp"
  out "as":string=" after test"
  out "bs":string
  out "bs":string="Humidity"
  out "as":string=" before test"
  out "bs":string="Humidity"
  out "S 61":string="Frictional Force ( N )"
  in  "Lan flag":dbl=22.0
  in  "Table":string[][](table)=[["ENGLISH TITLES", "RUSSIAN"], ["Winducom 2010", "Winducom  2010"], ["Exit", "Выход"], ["Acquire", "ИСПЫТАНИЕ     "], ["File Name :", "Имя файла :"], ["Sample ID :", "Имя образца :"], ["Remarks :", "Примечания :"], ["Standby", "ОЖИДАНИЕ"], ["Stop", "СТОП"], ["Frequency", "ЧАСТОТА"], ["Hz", "Гц"], ["Normal Load", "НАГРУЗКА"], ["N", "Н"], ["Temperature ( Deg C)", "ТЕМПЕРАТУРА (Град С)"], ["Heater On", "НАГРЕВ ВКЛ"], ["Humidity", "ВЛАЖНОСТЬ"], ["Rh", "%"], ["OFF", "ВЫКЛ"], ["Timer", "ВРЕМЯ"], ["Test duration", "ВРЕМЯ ТЕСТА"], ["min", "мин"], ["Elapsed Time", "依商判"], ["Save Dwell", "ИНТЕРВАЛ"], ["Sec", "Сек"], ["Count down ( Sec )", "До запуска (сек)"], ["Present ( Sec )", "Таймер (сек)"], ["Run", "Применить"], ["Power", "ПИТАНИЕ"], ["Test Status", "СТАТУС"], ["Manual Over Ride", "ПУСК"], ["Coefficient Of Friction", "КОЭФФИЦИЕНТ ТРЕНИЯ"], ["Data points", "Точки"], ["Reset Graph", "Сбросить график"], ["Frictional Force ( N )", "СИЛА ТРЕНИЯ (Н)"], ["ISO : WS1.4", "ISO : WS1.4"], ["Rh Before", "Влажность до"], ["Rh After", "Влажность, после"], ["Humidity, before test", "Влажность, до теста"], ["Humidity, after test", "Влажность, после теста"], ["Temp, before test", "Температура, до теста"], ["Temp, after test", "Температура, после теста"], ["AVP ", "СДП"], ["MWSD", "MWSD"], ["HCF", "ФКВ"], ["WS1.4", "WS1.4"], ["Save Result", "Сохранить результат"], ["COMPARE FILES", ""], ["File 1", "ФАЙЛ 1"], ["File 2", "ФАЙЛ 2"], ["File 3", "ФАЙЛ 3"], ["File 4", "ФАЙЛ 4"], ["Refresh", "ОБНОВИТЬ"], ["Coefficient Of Friction", "КОЭФФИЦИЕНТ ТРЕНИЯ"], ["Temperature", "ТЕМПЕРАТУРА"], ["Frictional Force ( N )", "СИЛА ТРЕНИЯ (Н)"], ["COF1", "КОФ1"], ["COF2", "КОФ2"], ["COF3", "КОФ3"], ["COF4", "КОФ4"], ["Reset Graph", "Сбросить график"], ["Time ( mins )", "Время (мин)"], ["Temperature ( Deg C)", "ТЕМПЕРАТУРА (Град С)"], ["Frictional  Force ( N )", "СИЛА ТРЕНИЯ (Н)"], ["ABOUT", ""], ["Frictional Force :", "КОЭФ.ТРЕНИЯ:"], ["Temperature :", "ТЕМПЕРАТУРА"], ["Speed Out:", "СКОРОСТЬ"], ["Air Temperature :", "ТЕМПЕРАТУРА ВОЗДУХА"], ["Humidity :", "ВЛАЖНОСТЬ"], ["Edit Gain Constant", "КОРРЕКТИРОВКА КОНСТАНТ"], ["Save Gain Constant", "СОХРАНИТЬ КОНСТАНТЫ"], ["Calibrate Parameter", "ПАРАМЕТРЫ КАЛИБРОВКИ"], ["Frictional Force ( N )", "СИЛА ТРЕНИЯ (Н)"], ["WINDUCOM 2010 \\XXXX\\VX.XX\\MONTH YEAR", "WINDUCOM 2010 \\XXXX\\VX.XX\\MONTH YEAR"], ["Stroke", "ДЛИННА ХОДА"], ["mm", "мм"], ["Air Temperature", "ВОЗДУХА ТЕМП"], ["Stroke", "ДЛИННА ХОДА "], ["Time ( mins )", "ВРЕМЯ ( мин )"], ["Sample Temperature( Deg C)", "Образец ТЕМПЕРАТУРА (Град С)"], ["Relative Humidity ( Rh )", "Относительный Влажность ( % )"], ["Air Temperature ( deg C )", "ТЕМПЕРАТУРА ВОЗДУХА (Град С)"], ["Save Gain Constants", "СОХРАНИТЬ КОНСТАНТЫ"], ["Password", "ПАРОЛЬ ДОСТУПА"], ["Enter Current Password", "ВВЕДИТЕ ТЕКУЩИЙ ПАРОЛЬ"], ["Enter The New Password", "ВВЕДИТЕ НОВЫЙ ПАРОЛЬ"], ["Change Calibrate Password", "Сбросить пароль калибровки"], ["Newtons ( N )", "Ньютон ( Н )"], ["File path", "Путь к файлу"], ["Threshold", "порог"], ["Run", "ПУСК"], ["Stop", "СТОП"], ["Displacement :", "смещение:"], ["Stroke Gain :", "ДЛИННА ХОДА:"], ["Port 1", "порт 1"], ["Port 2", "порт 2"], ["Ch-Power +:", "CH-ПИТАНИЕ +:"], ["Ch-Power -:", "CH-ПИТАНИЕ -:"], ["Ch-Heater:", "НАГРЕВ:"], ["Ch-Humidity Wet:", "CH-Увлажнение:"], ["Ch-Humidity Dry:", "CH-Осушение:"], ["Heater On", "НАГРЕВ ВКЛ"], ["Heater Off", "НАГРЕВ ВЫКЛ"], ["On", "ВКЛ"], ["Off", "ВЫКЛ"], ["TEXT REPORT", "ПРОТОКОЛ ИСПЫТАНИЯ"], ["Open Data File", "ОТКРЫТЬ ФАЙЛ ДАННЫХ"], ["Refresh", "ОБНОВЛЕНО"], ["Tittle", "заглавие"], ["Sample Design", "Образец"], ["Tested date", "Дата"], ["Sample ID ", "Имя образца"], ["Tested by", "Испытано"], ["System Configured Printers ", "Сконфигурированные принтеры"], ["Selected Printer", "Выбранный принтер"], ["Select Printer 3", "Выбрать  Печать"], ["Print", "Печать"], [":-@(WINDUCOM : RECIPROCATORY TEST RIG    DEFINITON FILE )      ", "(Анализатор HFRR с возвратно-поступательным механизмом для определения смазывающей способности дизельных топлив )"], ["Tested by:", "Оператор:"], ["          TIME;      COF;       STROKE  (mm);     AIR TEMP ( Deg C);  TEMP ( Deg C);  HUMIDITY ( Rh );", "КОЭФФИЦИЕНТ ТРЕНИЯ;   Инсульт; ТЕМПЕРАТУРА ВОЗДУХА; ВЛАЖНОСТЬ;"], ["Export", "Экспорт"], ["Temperature Intercept :", "ТЕМП перехват:"], ["Air Temperature Intercept:", "ТЕМП  ВОЗДУХА перехват:"], ["Select File Type ", "Выберете формат файла"], ["S.NO", "S.NO"], ["Trip", ""]]
  out "Residual Uno":string
  out "Residual Due":string
  out "String":string="C:\\Winducom 2010\\1582\\1582\\"
  out "file path":path=path "C:/Windows/wndcm_pw_stdED hfrr.txt"
  out "string":string="49\r50\r51\r10"
  out "x = y?":bool
  out "dipl pwd":string="@143$\n"
  out "string1 4":string
  out "string1 3":string
  out "string1 2":string
  out "string1":string
  out "stopT":bool
  out "Elapsed time 3":dbl=0.10620016403198242 min=0.0 max=6000.0 step=0.01 format="%<%H:%M:%S>t"
  in  "error in (no error)":errorcluster
  out "error out":errorcluster
  in  "RSTCOF 2":bool
  out "PID output":dbl=42.16277107130474 format="%.2f"
  out "Flag":dbl format="%.2f"
  in  "Tab Control 3":enum32{"RMS", "LIVE"}(tab)
  out "array w/ subset deleted":dbl[](array[numeric])
  out "REMARKS":string="@WINDUCOM : RECIPROCATORY TEST RIG    DEFINITON FILE       \r  Sample ID :- , Load :-  2.00 N , Remarks :- , Date :- 05/11/2016, 06:04\r"
  out "Time 2":dbl=0.0004
  in  "reinit":bool=TRUE
  in  "Remarks : 2":string
  out "PID-out":dbl
  out "Rate":dbl=2500.0 caption="Rate (Hz)" min=100.0 max=10000.0 step=1.0
  out "COUNT":i32
  out "FRICVALZ":dbl
  out "Sensor mean 3":dbl
  out "Sensor mean":dbl(slide) min=0.0 max=5.0 step=0.001 scale=0.0..5.0
  out "Sensor mean 2":dbl
  in  "ao0":errorcluster
  out "String 2":string
  out "clk":dbl min=0.0 max=999999999.0 step=0.25 format="%.2f"
  out "spm":string
  out "stp":dbl=0.25 min=0.25 max=60.0 step=0.25 format="%.2f"
  # "Step 4 — Calibration Result"
  # "© Copyright 2023 | Paltro Inc"
  # "HFRR ADV"
  # "ADV"
  # "Camera Initialization in Progress"
  # "Test Setup"
  # "SAMPLE INFO"
  # "Hz"
  # "grams"
  # "mm"
  # "°C"
  # "%RH"
  # "min"
  # "mins remaining"
  # "°C"
  # "Coefficient of Friction"
  # "Frictional Force ( N )"
  # "Electrical Contact Resistance ( % )"
  # "Temperature ( °C )"
  # "Heater"
  # "( mm )"
  # "Hz"
  # "%Rh"
  # "Stroke ( mm )"
  # "Controller"
  # "%"
  # "N"
  # "deg C"
  # "N"
  # "Automated Scar Detection in Progress"
  # "Zoom Factor"
  # "%"
  # "Tools"
  # "Wear Scar Measurements"
  # "Wear Scar"
  # "Wear Scar"
  # "Wear Scar"
  # "µm"
  # "µm"
  # "µm"
  # "Calibration Centre\nSelect a calibration procedure to begin. Each procedure guides you through all required steps."
  # "Apply known deadweight loads to validate \nthe friction force measurement chain \nand compute the calibration factor for the f\norce transducer."
  # "Step-by-step guided displacement calibration \nacross 12 positions from 0.1 mm to 1.2 mm. Tear \nfirst, then measure each position one by one."
  # "Two-set calibration: one point at 0 °C \nice-point) and one at 60 °C (high-point) \nusing a NIST-traceable reference resistor."
  # "Step 1 — Pre-calibration Setup"
  # "Prepare the displacement calibration reference gauge. Ensure the LVDT sensor is connected and the carriage slides freely. You will be guided through 6 positions from 0.2 mm to 1.2 mm, one at a time"
  # "Step 7 — Tare ( ZERO REFERENCE )"
  # "Before measuring, the sensor must be zeroed. Move the carriage to the mechanical zero stop — no displacement applied. Once in position, tap Tare & Begin to zero the reference."
  # "Step 8 — POSITION MEASUREMENT"
